vi "RSZVB Set Limit Response Domain Format Units.vi"(8 "error in (no error)":errorcluster {"code" format="%.0x"}, 9 "Response Units (0: Complex)":i32(ring) items=["Complex", "Magnitude", "Phase", "Real", "Imaginary", "SWR", "G Delay", "L", "C"], 10 "Channel (Trace) (1)":i32=1, 11 "VISA session":refnum<visa-resource-name>) -> (0 "error out":errorcluster {"code" format="%.0x"}, 3 "dup VISA session":refnum<visa-resource-name>)   [LabVIEW 2011]
doc: "This VI deletes the existing limit line and (re-)defines the physical units of the response values of the limit line.\n\nNotes: \n\n(1) This command is complemented by CALCulate<Chn>:LIMit:RDOMain:COMPlex and CALCulate<Chn>:LIMit:RDOMain:SPACing. \n\nRemote-control command(s):\nCALCulate<Chn>:LIMit:RDOMain:FORMat COMPlex | MAGNitude | PHASe | REAL | IMAGinary | SWR | GDELay | L | C"
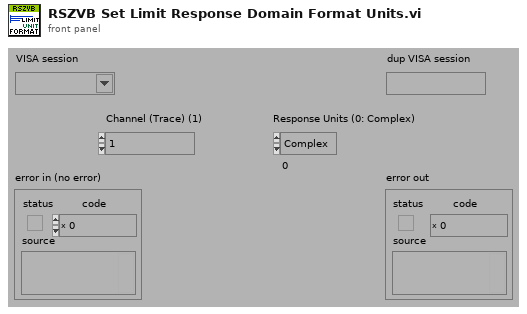
[diagram p1: front panel]
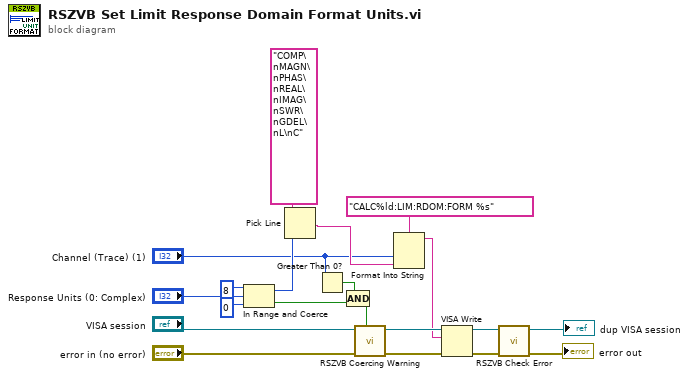
[diagram p0: block diagram]
diagram:
  n1 = In Range and Coerce(upper limit=8, x="Response Units (0: Complex)", lower limit=0) -> (coerced(x)=w10:i32, In Range?=w13:bool)
  n2 = Pick Line(multi-line string="COMP\nMAGN\nPHAS\nREAL\nIMAG\nSWR\nGDEL\nL\nC", line index=w10) -> (output string=w8:string)  [unwired: 1 in]
  n3 = Greater Than 0?(x="Channel (Trace) (1)") -> (x > 0?=w12:bool)
  n4 = Compound Arithmetic op=AND(w12, w13) -> (w11:bool)
  n5 = call "RSZVB Coercing Warning.vi"("In Range?"=w11, "error in (no error)"="error in (no error)", "VISA session"="VISA session") -> ("error out"=w19:errorcluster, "dup VISA session"=w20:refnum<visa-resource-name>)  [unwired: 7 in]
  n6 = Format Into String(format string="CALC%ld:LIM:RDOM:FORM %s", "Channel (Trace) (1)", w8) -> (resulting string=w16:string)  [unwired: 2 in, 1 out]
  n7 = VISA Write(VISA resource name=w20, write buffer=w16, error in (no error)=w19) -> (VISA resource name out=w17:refnum<visa-resource-name>, error out=w18:errorcluster)  [unwired: 1 out]
  n8 = call "RSZVB Check Error.vi"("error in (no error)"=w18, "VISA session"=w17) -> ("error out"=→"error out":errorcluster, "dup VISA session"=→"dup VISA session":refnum<visa-resource-name>)  [unwired: 8 in]
